vi "ques 3.vi"() -> ()   [LabVIEW 2022 SP3]
panel:
  in  "Filename":path=path "C:/Users/rohan/OneDrive/Desktop/VI LAB/Assignment 5/New.lvm"
  out "Time":string
  out "Date":string
  # "Aditya Singh\n    2315005"
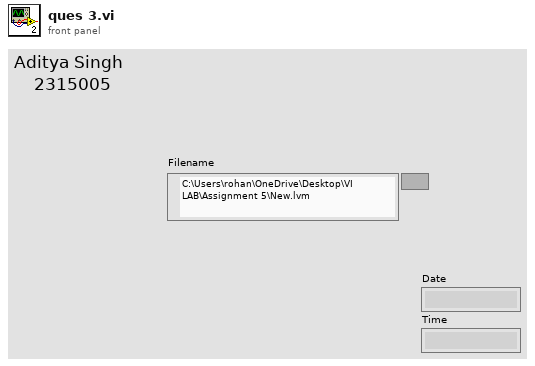
[diagram p1: front panel]
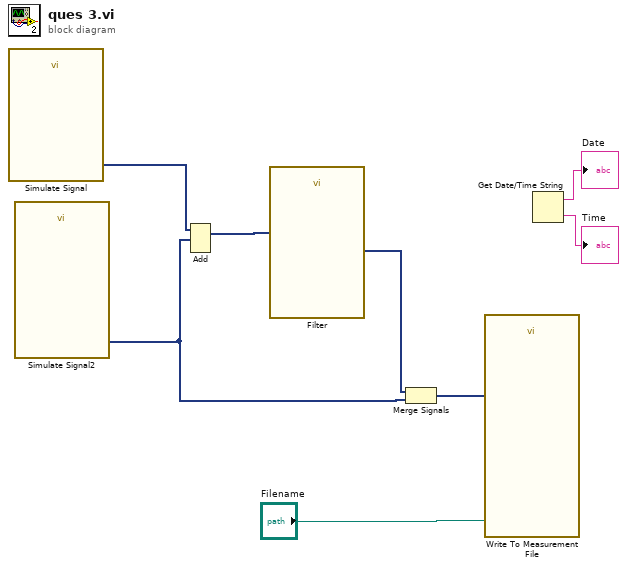
[diagram p0: block diagram]
diagram:
  n1 = call "Simulate Signal"() -> ("Sine"=w8:dynamicdata)  [unwired: 14 in, 1 out]
  n2 = call "Simulate Signal2"() -> ("Square"=w3:dynamicdata)  [unwired: 14 in, 1 out]
  n3 = Add(1:w3, 2:w8) -> (0:w7:dynamicdata)  [unwired: 1 in, 1 out]
  n4 = call "Filter"("Signal"=w7) -> ("Filtered Signal"=w4:dynamicdata)  [unwired: 9 in, 1 out]
  n5 = Merge Signals(w4, w3) -> (w2:dynamicdata)
  n6 = call "Write To Measurement File"("Signals"=w2, "Filename"="Filename") -> ()  [unwired: 15 in, 3 out]
  n7 = Get Date/Time String() -> (date string=→"Date":string, time string=→"Time":string)  [unwired: 3 in]
